vi "Gestione cluster allarmi.vi"(0 "serial master instance":refnum<class "Modbus Master.lvclass">, 1 "Cluster ALARMS":refnum<vi>, 5 "Array Name alarms":string[](array[string]), 7 "Boolean array":bool[](array[boolean]), 9 "Array descriz alarms":string[](array[string]), 11 "error in (no error)":errorcluster) -> (4 "Modbus master out":refnum<class "Modbus Master.lvclass">, 15 "error out":errorcluster)   [LabVIEW 2019]
uses:
  <vilib>/Modbus/master/Modbus Master.lvclass
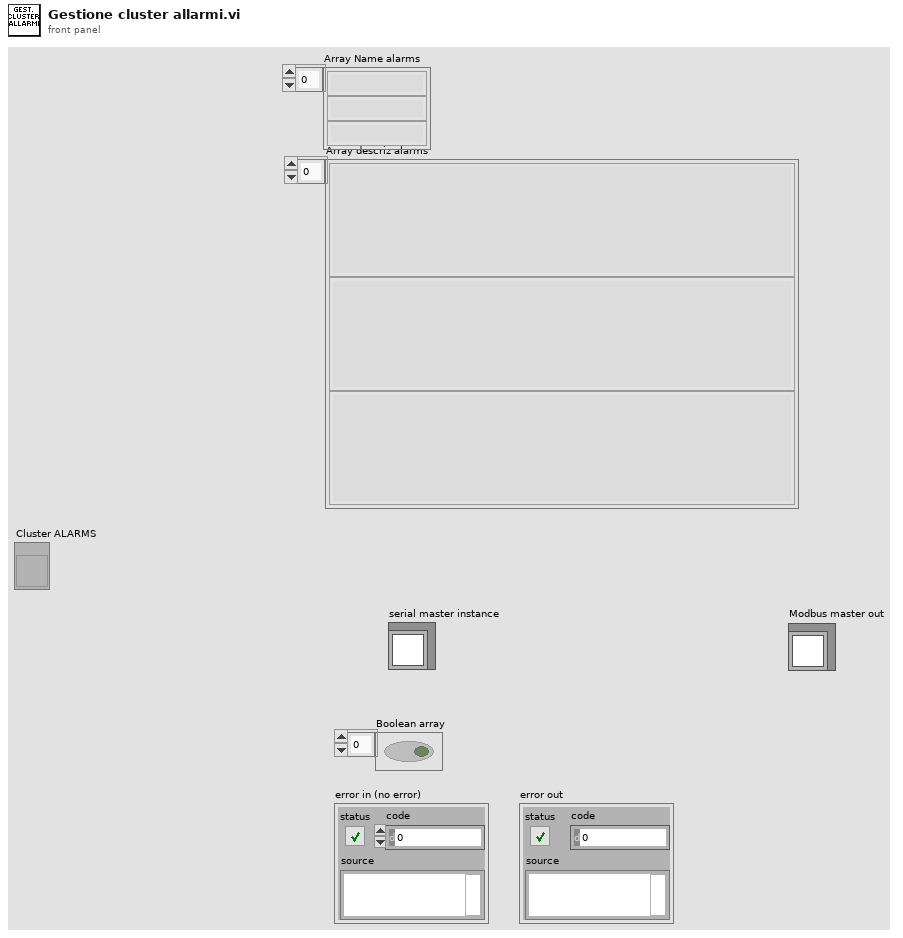
[diagram p1: front panel]
types:
  T1 = cluster{"ALARMS":cluster{"A 00":bool, "A 01":bool, "A 02":bool, "A 03":bool, "A 04":bool, "A 05":bool, "A 06":bool, "A 07":bool, "A 08":bool, "A 09":bool, "A 10":bool, "A 11":bool, "A 12":bool, "A 13":bool, "A 14":bool, "A 15":bool}, "DISABLE":cluster{"A 00":bool, "A 1":bool, "A 2":bool, "A 3":bool, "A 4":bool, "A 5":bool, "A 6":bool, "A 7":bool, "A 8":bool, "A 9":bool, "A 10":bool, "A 11":bool, "A 12":bool, "A 13":bool, "A 14":bool, "A 15":bool}, "NAME":string[], "SUBCODE>DESCRIPTION":string[]}
  T2 = cluster{"Boolean array[0]":bool, "Boolean array[1]":bool, "Boolean array[2]":bool, "Boolean array[3]":bool, "Boolean array[4]":bool, "Boolean array[5]":bool, "Boolean array[6]":bool, "Boolean array[7]":bool, "Boolean array[8]":bool, "Boolean array[9]":bool, "Boolean array[10]":bool, "Boolean array[11]":bool, "Boolean array[12]":bool, "Boolean array[13]":bool, "Boolean array[14]":bool, "Boolean array[15]":bool}
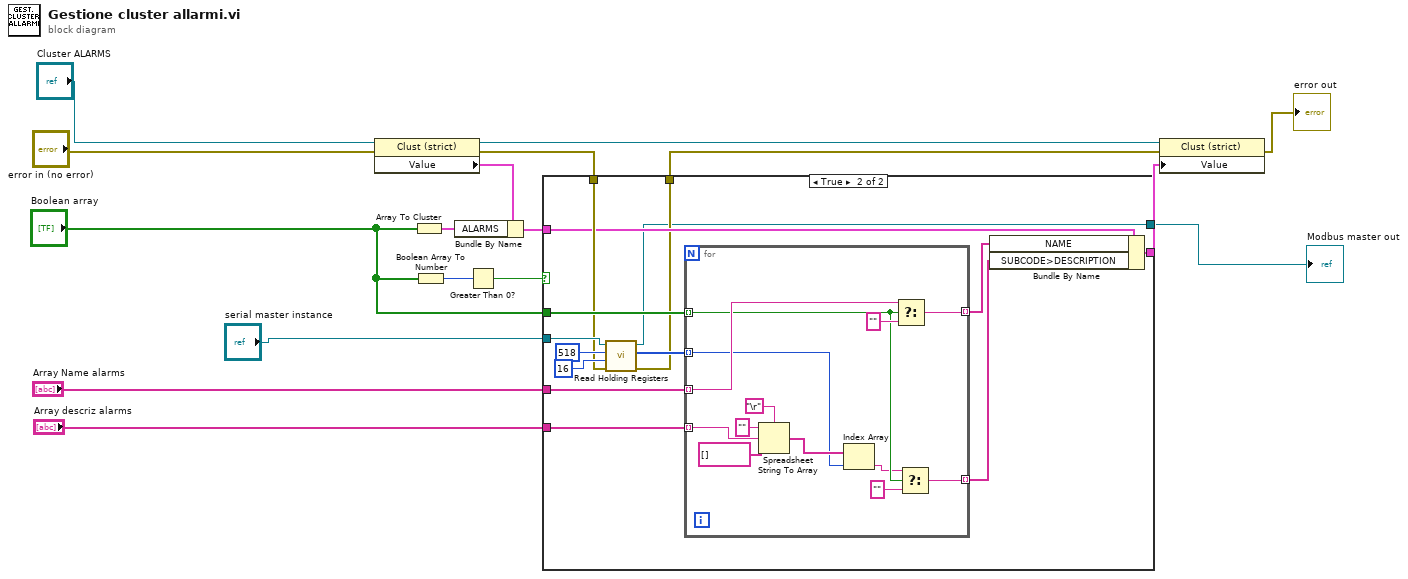
[diagram p0: block diagram]
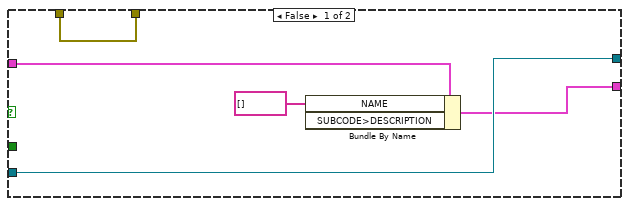
[diagram p2: hidden frame]
diagram:
  n1 = property class="Clust (strict)"(reference="Cluster ALARMS", error in="error in (no error)") -> (reference out=w6:refnum<vi>, error out=w7:errorcluster, "Value"=w16:T1)
  n2 = Array To Cluster(array="Boolean array") -> (cluster=w17:T2)
  n3 = Boolean Array To Number(Boolean array="Boolean array") -> (number=w14:u32)
  n4 = Bundle By Name(cluster=w16, "ALARMS"=w17) -> (w10:T1)
  n5 = Greater Than 0?(x=w14) -> (x > 0?=w13:bool)
  n6 = case shown="True" w13 {
    tunnel: "Array Name alarms" -> [_ w36]
    tunnel: "Boolean array" -> [_ w35]
    tunnel: w10 -> [w21 w28]
    tunnel: "Array descriz alarms" -> [_ w34]
    tunnel: "serial master instance" -> [w22 w32]
    tunnel: w7 -> [w18 w29]
    tunnel: [w20 w25] -> w5
    tunnel: [w18 w24] -> w4
    tunnel: [w22 w23] -> w3
    frame False {
      w19 = string[] [] ("NAME")
      n7 = Bundle By Name(cluster=w21, "NAME"=w19, "SUBCODE>DESCRIPTION"=w19) -> (w20:T1)
    }
    frame True {
      n8 = call-dynamic "Read Holding Registers.vi"("error in (no error)"=w29, "number of holding registers"=u16 16, "starting address"=u16 518, "Modbus master in"=w32) -> ("error out"=w24:errorcluster, "register values"=w30:u16[], "Modbus master out"=w23:refnum<class "Modbus Master.lvclass">)  [unwired: 5 in]
      n9 = for {
        tunnel: w36 -> [w49] mode=indexing
        tunnel: w35 -> [w43] mode=indexing
        tunnel: [w47] -> w27 mode=indexing
        tunnel: w34 -> [w46] mode=indexing
        tunnel: [w40] -> w26 mode=indexing
        tunnel: w30 -> [w39] mode=indexing
        n10 = Spreadsheet String To Array(delimiter (Tab)="\r", format string="", spreadsheet string=w46, array type (2D Dbl)=string[] [] ("Array descriz alarms")) -> (array=w42:string[])
        n11 = Index Array(array=w42, index=w39) -> (element=w41:string)
        n12 = Select(t=w49, s=w43, f="") -> (s? t:f=w47:string)
        n13 = Select(t=w41, s=w43, f="") -> (s? t:f=w40:string)
      }
      n14 = Bundle By Name(cluster=w28, "NAME"=w27, "SUBCODE>DESCRIPTION"=w26) -> (w25:T1)
    }
  }
  "Modbus master out" <- w3
  n15 = property class="Clust (strict)"(reference=w6, error in=w4, "Value"=w5) -> (error out=→"error out":errorcluster)  [unwired: 1 out]
